vi "总磷总氮公式写入.vi"(7 "公式":cluster{"X^2":dbl, "X":dbl, "b":dbl}, 8 "error in (no error)":errorcluster caption="错误输入（无错误）", 9 "量程":enum16{"低量程", "高量程"}(ring), 10 "测量模式":enum16{"水样测量", "零点核查", "跨度核查", "标样核查", "加标回收"}(ring), 11 "测量参数":u16(ring) items=["总磷"=1, "总氮"=2, "氨氮"=3, "COD"=22]) -> (0 "error out":errorcluster caption="错误输出")   [LabVIEW 2016, in "斯坦道总氮.lvlib"]
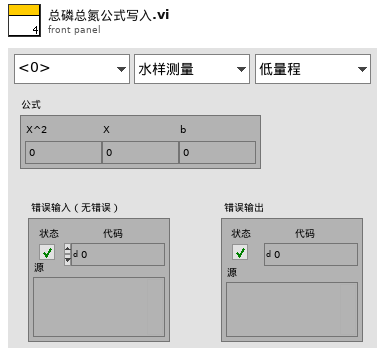
[diagram p1: front panel]
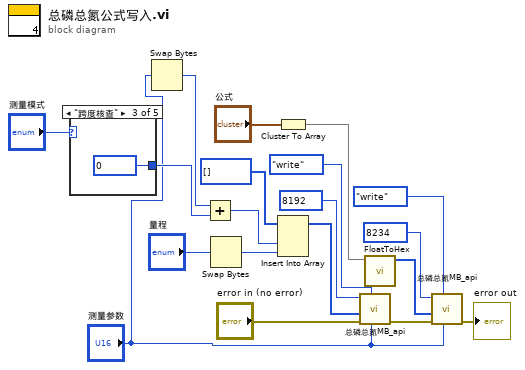
[diagram p0: block diagram]
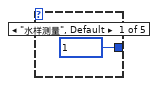
[diagram p2: hidden frame]
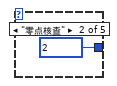
[diagram p3: hidden frame]
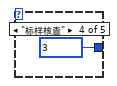
[diagram p4: hidden frame]
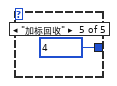
[diagram p5: hidden frame]
diagram:
  n1 = case shown="\"跨度核查\"" "测量模式" {
    tunnel: [u16 1 ("starting address") u16 2 ("starting address") u16 0 ("starting address") u16 3 ("starting address") u16 4 ("starting address")] -> w5
    frame "水样测量", Default {
    }
    frame "零点核查" {
    }
    frame "跨度核查" {
    }
    frame "标样核查" {
    }
    frame "加标回收" {
    }
  }
  n2 = Swap Bytes(anything="测量参数") -> (byte swapped=w3:u16)
  n3 = Add(x=w3, y=w5) -> (x+y=w13:u16)
  n4 = Swap Bytes(anything="量程") -> (byte swapped=w1:u16)
  n5 = Cluster To Array(cluster="公式") -> (array=w18:dbl[])
  n6 = Insert Into Array(array=u16[] [] ("数组"), new element #1=w13, new element #2=w1) -> (w7:u16[])  [unwired: 1 in]
  n7 = call "总磷总氮MB_api.vi"("Slave ID"="测量参数", "STEP"=enum16{"open", "read", "write", "close"}."write", "Error in"="error in (no error)", "values"=w7, "starting address"=u16 8192) -> ("error out"=w10:errorcluster)  [unwired: 4 in, 2 out]
  n8 = call "FloatToHex.vi"("浮点数"=w18) -> ("DCBA整形输出"=w6:u16[])  [unwired: 10 in]
  n9 = call "总磷总氮MB_api.vi"("Slave ID"="测量参数", "STEP"=enum16{"open", "read", "write", "close"}."write", "Error in"=w10, "values"=w6, "starting address"=u16 8234) -> ("error out"=→"error out":errorcluster)  [unwired: 4 in, 2 out]
